vi "Repeat_ERD_Read.vi"(0 "GEA2 Reference In":refnum<k24>, 1 "GEA Inputs":T4 {"Destination" format="%.0x"; "Source" format="%.0x"}, 2 "Standalone?":bool, 11 "Error In":errorcluster, 12 "Repeat Count":i32, 13 "Read ERD List":T2[](array[typedef]) {"ERD Number" format="%.0x"}) -> (4 "GEA2 Reference Out":refnum<k24>, 8 "ERD Data Out":T1[](array[typedef]) {"ERD Number" format="%.0x"}, 10 "Raw Data Out":string, 15 "Error Out":errorcluster)   [LabVIEW 2016, in "Centauro.lvlib"]
doc: "This vi can be used to read ERD every 1 sec for user selected repeat counts."
uses:
  Projects/Centauro.lvlib
  Q:/Common/DLLs/GEA3/GeaCommunication.dll
  Common/DLLs/GEA3/GeaCommunication.dll
  Common/LabVIEW GEA2 Toolkit/LabVIEW_GEA2_Toolkit.lvlibp/type defs/Source_Destination.ctl
  Common/LabVIEW GEA2 Toolkit/LabVIEW_GEA2_Toolkit.lvlibp/type defs/ERD Read Data In.ctl
  Common/LabVIEW GEA2 Toolkit/LabVIEW_GEA2_Toolkit.lvlibp/type defs/Data Type.ctl
  Common/LabVIEW GEA2 Toolkit/LabVIEW_GEA2_Toolkit.lvlibp/type defs/ERD Read Data Out.ctl
  Common/LabVIEW GEA2 Toolkit/LabVIEW_GEA2_Toolkit.lvlibp
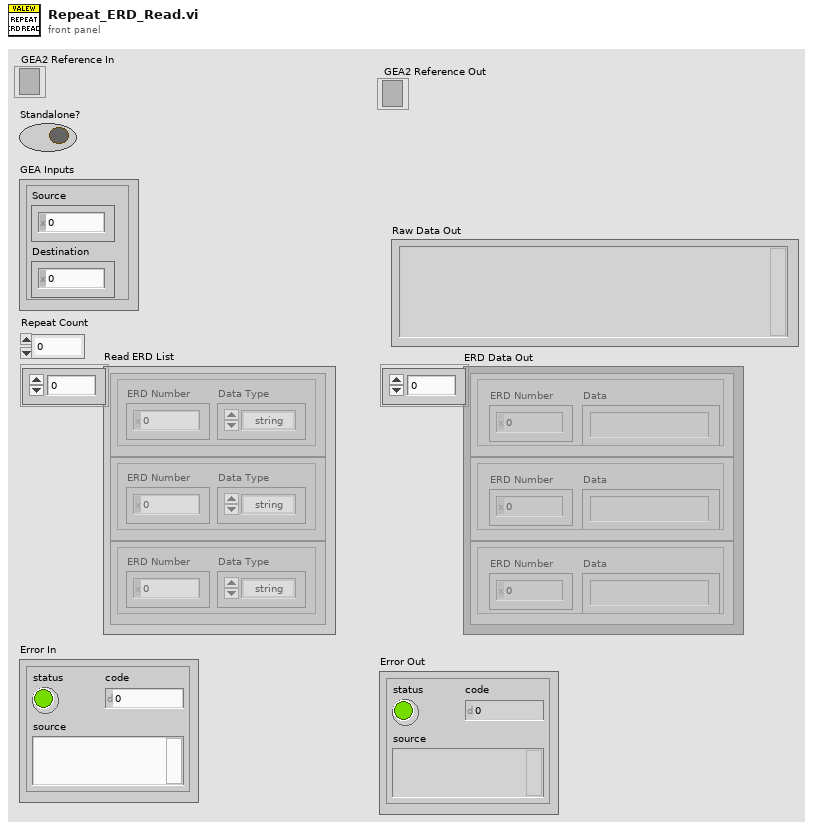
[diagram p1: front panel]
types:
  T1 = typedef "LabVIEW_GEA2_Toolkit.lvlibp/ERD Read Data Out.ctl" = cluster{"ERD Number":u16, "Data":string}
  T2 = typedef "LabVIEW_GEA2_Toolkit.lvlibp/ERD Read Data In.ctl" = cluster{"ERD Number":u16, "Data Type":T3}
  T3 = typedef "LabVIEW_GEA2_Toolkit.lvlibp/Data Type.ctl" = enum16{"string", "boolean", "uint8_t", "uint16_t", "uint32_t", "uint64_t", "int8_t", "int16_t", "int32_t", "int64_t"}
  T4 = typedef "LabVIEW_GEA2_Toolkit.lvlibp/Source_Destination.ctl" = cluster{"Source":u8, "Destination":u8}
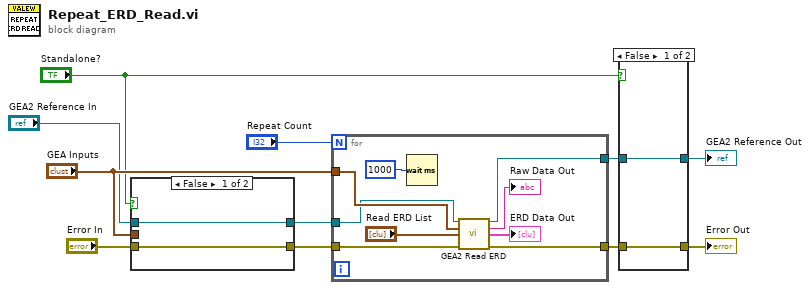
[diagram p0: block diagram]
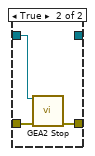
[diagram p2: hidden frame]
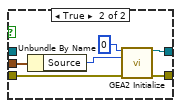
[diagram p3: hidden frame]
diagram:
  n1 = case shown="False" "Standalone?" {
    tunnel: "Error In" -> [w12 w19]
    tunnel: [w12 w18] -> w6
    tunnel: "GEA2 Reference In" -> [w13 _]
    tunnel: [w13 w17] -> w5
    tunnel: "GEA Inputs" -> [_ w15]
    frame False {
    }
    frame True {
      n2 = Unbundle By Name(w15) -> ("Source"=w16:u8)
      n3 = call "GEA2 Initialize.vi"("Board Index"=0, "Source Address"=w16, "error in"=w19) -> ("GEA2 Reference Out"=w17:refnum<k24>, "error out"=w18:errorcluster)  [unwired: 10 in, 1 out]
    }
  }
  n4 = for {
    N: "Repeat Count" -> [_]
    tunnel: "GEA Inputs" -> [w28]
    tunnel: [w20] -> w2
    tunnel: [w27] -> w1
    tunnel: w5 -> [w26]
    tunnel: w6 -> [w25]
    n5 = Wait (ms)(milliseconds to wait=u32 1000) -> ()  [unwired: 1 out]
    n6 = call "GEA2 Read ERD.vi"("GEA2 Reference In"=w26, "GEA Inputs"=w28, "Read ERD List"="Read ERD List", "Error In"=w25) -> ("GEA2 Reference Out"=w27:refnum<k24>, "Raw Data Out"=→"Raw Data Out":string, "ERD Data Out"=→"ERD Data Out":T1[], "Error Out"=w20:errorcluster)  [unwired: 8 in]
  }
  n7 = case shown="False" "Standalone?" {
    tunnel: w2 -> [w29 w32]
    tunnel: [w29 w31] -> w10
    tunnel: w1 -> [w30 w33]
    tunnel: [w30 _] -> w4
    frame False {
    }
    frame True {
      n8 = call "GEA2 Stop.vi"("GEA2 Reference In"=w33, "Error In"=w32) -> ("Error Out"=w31:errorcluster)  [unwired: 13 in]
    }
  }
  "Error Out" <- w10
  "GEA2 Reference Out" <- w4
